vi "saveTestParameters.vi"(8 "error in (no error)":errorcluster, 11 "Logger in":refnum<class "TestDataLog.lvclass">) -> (0 "error out":errorcluster, 3 "Logger out":refnum<class "TestDataLog.lvclass">)   [LabVIEW 2013, in "TestDataLog.lvclass"]
uses:
  TestDataLog.lvclass
  <userlib>/Common/Log/Log/Log.lvclass/Log.ctl
  TestDataLog.lvclass/TestDataLog.ctl
  <userlib>/Common/Log/Log/Log.lvclass
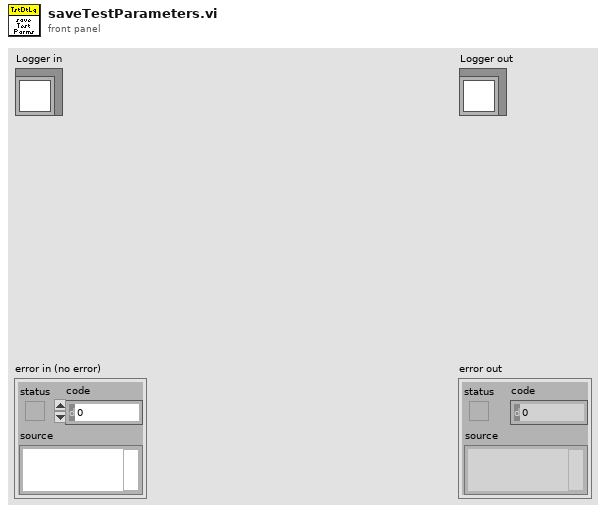
[diagram p1: front panel]
types:
  T1 = typedef "TestParameters.ctl" = cluster{"Number of cycles for complete test":u32, "Cycle profile":T2, "PGA Gain Coefficients":u8[], "Temperature Transition Wait Time":dbl[unit], "Temperature Settled StDev":dbl[unit], "Temperature Settling Sample Size":u16, "Bridge Measurement Sample Size":u16}
  T2 = typedef "CycleProfileConfig.ctl" = cluster{"Temperature Setpoint":dbl[unit][], "Soak Time":dbl[unit][], "Gain Stabilization Time":dbl[unit][], "Pause After Step":dbl[unit][]}
  T3 = typedef "Log.lvlib/Log.ctl" = cluster{"Log Directory":path, "Log Filename Base":string, "Max records per file":u32, "Comment":string}
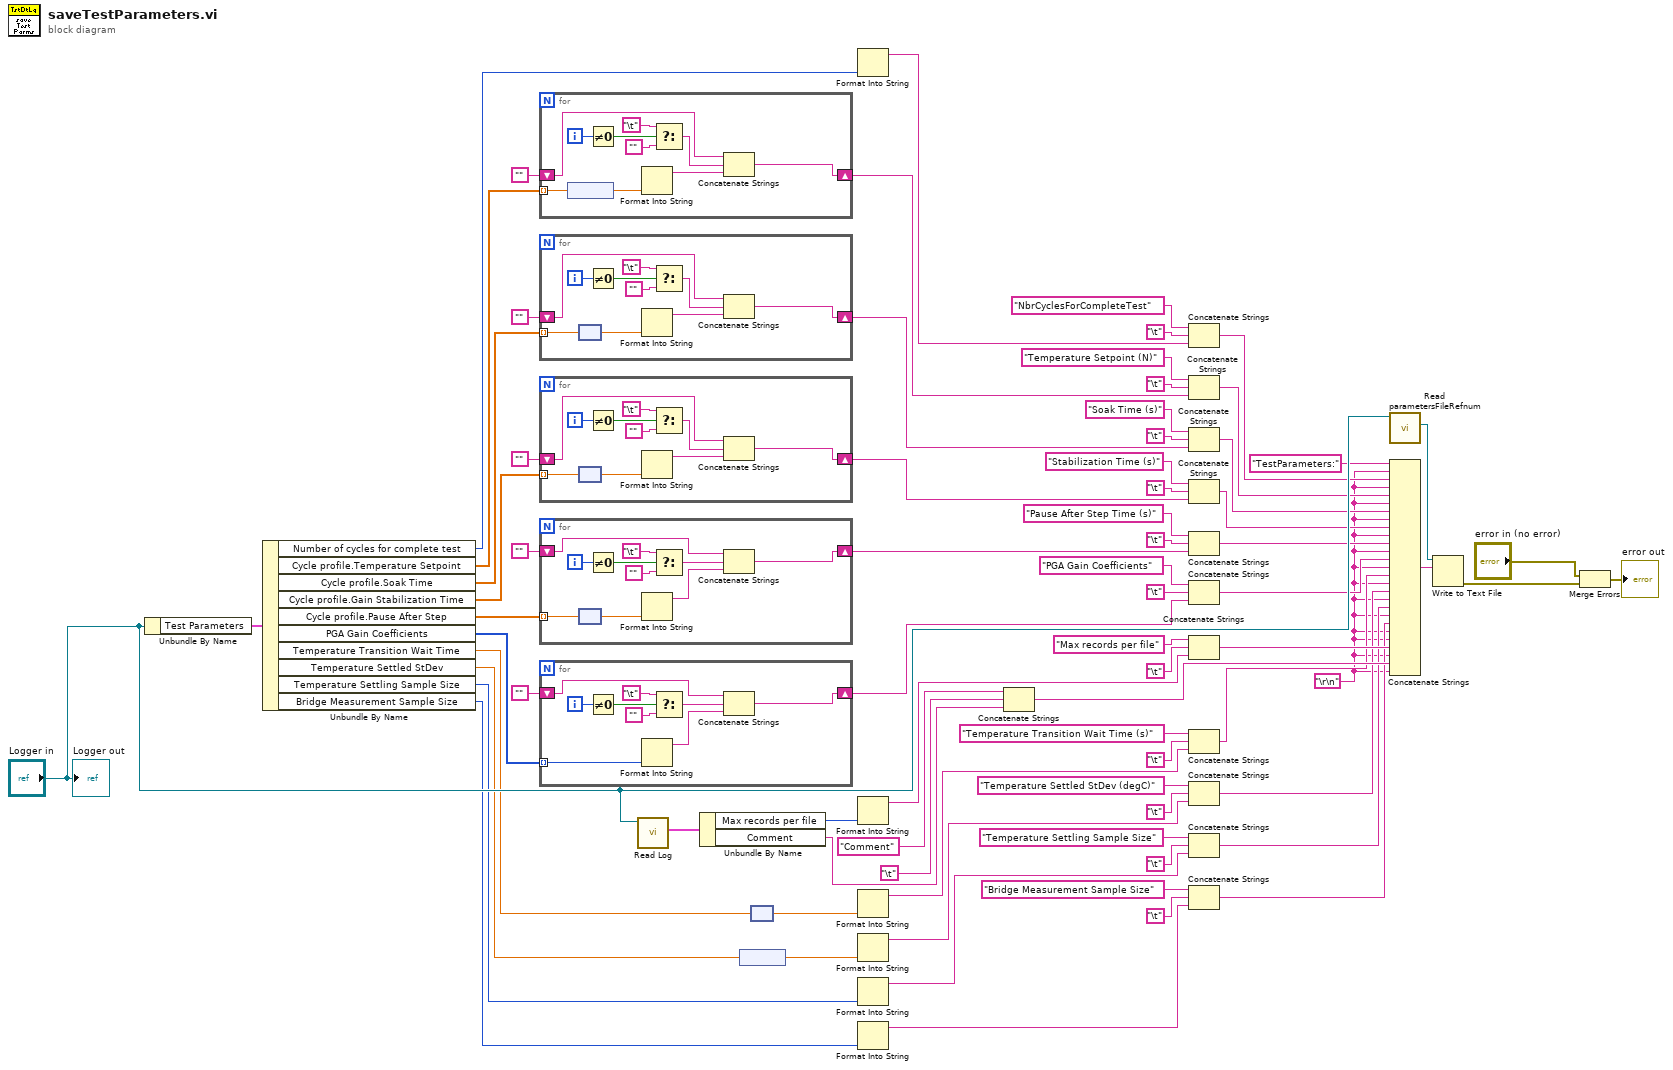
[diagram p0: block diagram]
diagram:
  w5 = "\r\n"
  n1 = Unbundle By Name("Logger in") -> ("Test Parameters"=w76:T1)
  n2 = Unbundle By Name(w76) -> ("Number of cycles for complete test"=w75:u32, "Cycle profile.Temperature Setpoint"=w74:dbl[unit][], "Cycle profile.Soak Time"=w72:dbl[unit][], "Cycle profile.Gain Stabilization Time"=w33:dbl[unit][], "Cycle profile.Pause After Step"=w32:dbl[unit][], "PGA Gain Coefficients"=w25:u8[], "Temperature Transition Wait Time"=w2:dbl[unit], "Temperature Settled StDev"=w4:dbl[unit], "Temperature Settling Sample Size"=w9:u16, "Bridge Measurement Sample Size"=w8:u16)
  n3 = for {
    tunnel: w74 -> [w81] mode=indexing
    shift-right: [w86] -> w60
    shift-left: "" -> [w85]
    i -> [w84]
    n4 = node(w81) -> (w80:dbl)
    n5 = Not Equal To 0?(x=w84) -> (x != 0?=w83:bool)
    n6 = Format Into String(w80) -> (resulting string=w82:string)  [unwired: 3 in, 1 out]
    n7 = Select(t="\t", s=w83, f="") -> (s? t:f=w77:string)
    n8 = Concatenate Strings(w85, w77, w82) -> (w86:string)
  }
  n9 = for {
    tunnel: w72 -> [w91] mode=indexing
    shift-right: [w96] -> w56
    shift-left: "" -> [w95]
    i -> [w94]
    n10 = node(w91) -> (w90:dbl)
    n11 = Not Equal To 0?(x=w94) -> (x != 0?=w93:bool)
    n12 = Format Into String(w90) -> (resulting string=w92:string)  [unwired: 3 in, 1 out]
    n13 = Select(t="\t", s=w93, f="") -> (s? t:f=w87:string)
    n14 = Concatenate Strings(w95, w87, w92) -> (w96:string)
  }
  n15 = for {
    tunnel: w33 -> [w101] mode=indexing
    shift-right: [w106] -> w41
    shift-left: "" -> [w105]
    i -> [w104]
    n16 = node(w101) -> (w100:dbl)
    n17 = Not Equal To 0?(x=w104) -> (x != 0?=w103:bool)
    n18 = Format Into String(w100) -> (resulting string=w102:string)  [unwired: 3 in, 1 out]
    n19 = Select(t="\t", s=w103, f="") -> (s? t:f=w97:string)
    n20 = Concatenate Strings(w105, w97, w102) -> (w106:string)
  }
  n21 = for {
    tunnel: w32 -> [w111] mode=indexing
    shift-right: [w116] -> w34
    shift-left: "" -> [w115]
    i -> [w114]
    n22 = node(w111) -> (w110:dbl)
    n23 = Not Equal To 0?(x=w114) -> (x != 0?=w113:bool)
    n24 = Format Into String(w110) -> (resulting string=w112:string)  [unwired: 3 in, 1 out]
    n25 = Select(t="\t", s=w113, f="") -> (s? t:f=w107:string)
    n26 = Concatenate Strings(w115, w107, w112) -> (w116:string)
  }
  n27 = for {
    tunnel: w25 -> [w117] mode=indexing
    shift-right: [w125] -> w24
    shift-left: "" -> [w124]
    i -> [w123]
    n28 = Not Equal To 0?(x=w123) -> (x != 0?=w122:bool)
    n29 = Format Into String(w117) -> (resulting string=w121:string)  [unwired: 3 in, 1 out]
    n30 = Select(t="\t", s=w122, f="") -> (s? t:f=w118:string)
    n31 = Concatenate Strings(w124, w118, w121) -> (w125:string)
  }
  n32 = call <userlib>:"Read Log.vi"("Log in"="Logger in") -> ("Log"=w70:T3)  [unwired: 9 in, 1 out]
  n33 = Unbundle By Name(w70) -> ("Max records per file"=w69:u32, "Comment"=w49:string)
  n34 = node(w4) -> (w3:dbl)
  n35 = node(w2) -> (w1:dbl)
  n36 = Format Into String(w75) -> (resulting string=w63:string)  [unwired: 3 in, 1 out]
  n37 = Format Into String(w69) -> (resulting string=w51:string)  [unwired: 3 in, 1 out]
  n38 = Format Into String(w1) -> (resulting string=w21:string)  [unwired: 3 in, 1 out]
  n39 = Format Into String(w3) -> (resulting string=w19:string)  [unwired: 3 in, 1 out]
  n40 = Format Into String(w9) -> (resulting string=w15:string)  [unwired: 3 in, 1 out]
  n41 = Format Into String(w8) -> (resulting string=w12:string)  [unwired: 3 in, 1 out]
  n42 = Concatenate Strings("Comment" ("element"), "\t", w49) -> (w47:string)
  n43 = Concatenate Strings("NbrCyclesForCompleteTest" ("element"), "\t", w63) -> (w65:string)
  n44 = Concatenate Strings("Temperature Setpoint (N)" ("element"), "\t", w60) -> (w59:string)
  n45 = Concatenate Strings("Soak Time (s)" ("element"), "\t", w56) -> (w55:string)
  n46 = Concatenate Strings("Stabilization Time (s)" ("element"), "\t", w41) -> (w31:string)
  n47 = Concatenate Strings("Pause After Step Time (s)" ("element"), "\t", w34) -> (w30:string)
  n48 = Concatenate Strings("PGA Gain Coefficients" ("element"), "\t", w24) -> (w27:string)
  n49 = Concatenate Strings("Max records per file" ("element"), "\t", w51) -> (w48:string)
  n50 = Concatenate Strings("Temperature Transition Wait Time (s)" ("element"), "\t", w21) -> (w20:string)
  n51 = Concatenate Strings("Temperature Settled StDev (degC)" ("element"), "\t", w19) -> (w16:string)
  n52 = Concatenate Strings("Temperature Settling Sample Size" ("element"), "\t", w15) -> (w7:string)
  n53 = Concatenate Strings("Bridge Measurement Sample Size" ("element"), "\t", w12) -> (w6:string)
  n54 = call <userlib>:"Read parametersFileRefnum.vi"("Log in"="Logger in") -> ("parametersFileRefnum"=w46:refnum<file>)  [unwired: 9 in, 1 out]
  n55 = Concatenate Strings("TestParameters:", w5, w65, w5, w59, w5, w55, w5, w31, w5, w30, w5, w27, w5, w20, w5, w16, w5, w7, w5, w6, w5, w5, w48, w5, w47, w5) -> (w45:string)
  n56 = Write to Text File(file (use dialog)=w46, text=w45) -> (error out=w43:errorcluster)  [unwired: 2 in, 2 out]
  n57 = Merge Errors("error in (no error)", w43) -> (→"error out":errorcluster)
  "Logger out" <- "Logger in"
